vi "addTxBuffer.vi"(8 "error in (no error)":errorcluster, 10 "Frame":T1 {"Data" format="%02x"}, 11 "Modbus in":refnum<class "Modbus.lvclass">) -> (0 "error out":errorcluster, 3 "Modbus out":refnum<class "Modbus.lvclass">)   [LabVIEW 2015, in "RTModbus.lvlib" / "Modbus.lvclass"]
uses:
  Modbus.lvclass
  DataTypes/Frame.ctl
  Modbus.lvclass/Modbus.ctl
  RTModbus.lvlib
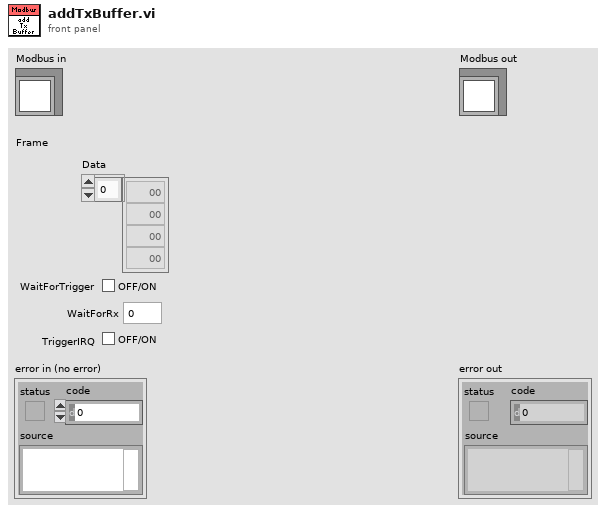
[diagram p1: front panel]
types:
  T1 = typedef "RTModbus.lvlib/Frame.ctl" = cluster{"Data":u8[], "WaitForTrigger":bool, "WaitForRx":u16, "TriggerIRQ":bool}
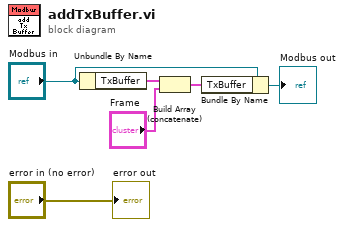
[diagram p0: block diagram]
diagram:
  n1 = Unbundle By Name("Modbus in") -> ("TxBuffer"=w6:T1[])
  n2 = Build Array (concatenate)(w6, "Frame") -> (w2:T1[])
  n3 = Bundle By Name(cluster="Modbus in", "TxBuffer"=w2) -> (→"Modbus out":refnum<class "Modbus.lvclass">)
  "error out" <- "error in (no error)"
